vi "Open.vi"(8 "error in (no error)":errorcluster, 11 "UDP in":refnum<class "UDP.lvclass">) -> (0 "error out":errorcluster, 3 "UDP out":refnum<class "UDP.lvclass">)   [LabVIEW 2018, in "UDP.lvclass"]
doc: "Bus.lvclass:Open.vi\n\nThis is the template for the Open VI for the Bus class.\n\nInstrument Communication Module Version 1.0\nJuly, 2017 Original Code Consulting David Thomson\n www.originalcode.com"
uses:
  UDP.lvclass
  UDP.lvclass/UDP.ctl
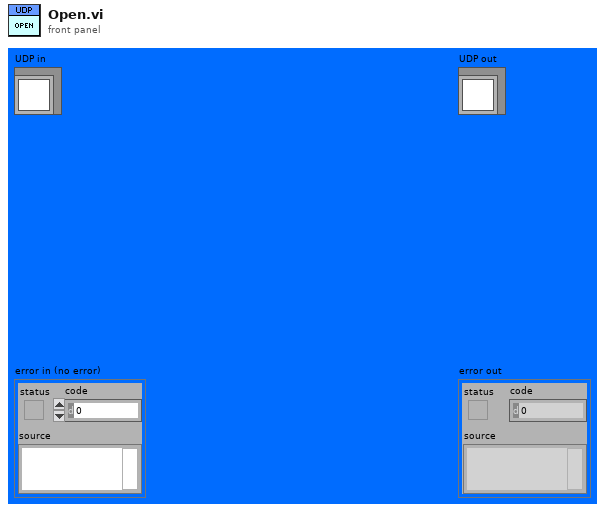
[diagram p1: front panel]
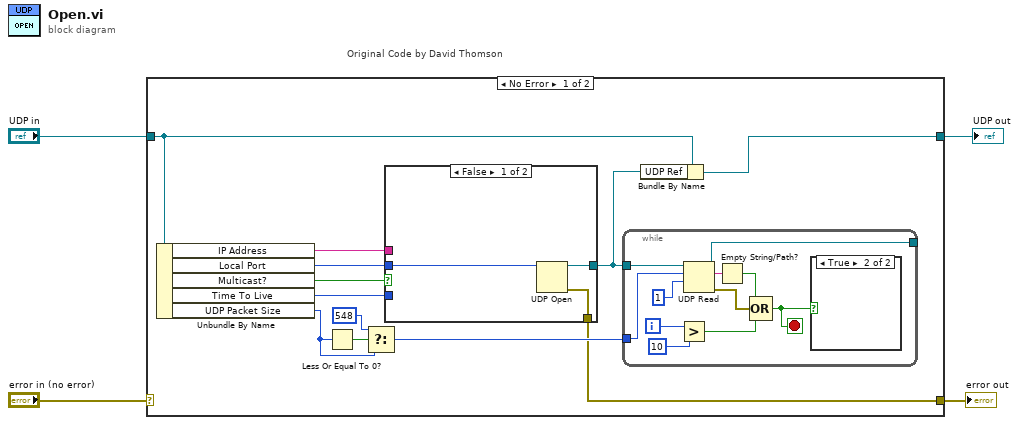
[diagram p0: block diagram]
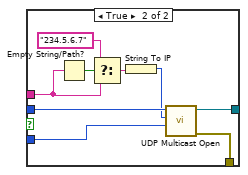
[diagram p2: hidden frame]
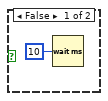
[diagram p3: hidden frame]
diagram:
  n1 = case "Original Code by David Thomson" shown="No Error" "error in (no error)" {
    selector: "error in (no error)" -> [_ w42]
    tunnel: [w11 w42] -> w1
    tunnel: [w6 w41] -> w2
    tunnel: "UDP in" -> [w7 w41]
    frame No Error {
      n2 = Unbundle By Name(w7) -> ("IP Address"=w9:string, "Local Port"=w16:u16, "Multicast?"=w10:bool, "Time To Live"=w8:u16, "UDP Packet Size"=w13:i32)
      n3 = Less Or Equal To 0?(x=w13) -> (x <= 0?=w15:bool)
      n4 = Select(t=548 ("max size (548)"), s=w15, f=w13) -> (s? t:f=w12:i32)
      n5 = case shown="False" w10 {
        tunnel: w16 -> [w19 w26]
        tunnel: [w18 w28] -> w5
        tunnel: [w17 w27] -> w11
        tunnel: w9 -> [_ w22]
        tunnel: w8 -> [_ w20]
        frame False {
          n6 = UDP Open(11:w19) -> (port=w18:refnum<k16>, 0:w17:errorcluster)  [unwired: 1 in, 4 out]
        }
        frame True {
          n7 = Empty String/Path?(string/path=w22) -> (empty?=w25:bool)
          n8 = Select(t="234.5.6.7", s=w25, f=w22) -> (s? t:f=w24:string)
          n9 = String To IP(1:w24) -> (0:w21:u32)
          n10 = call-poly "UDP Multicast Open.vi"("time-to-live (1)"=w20, "multicast addr"=w21, "port"=w26) -> ("error out"=w27:errorcluster, "connection ID"=w28:refnum<k16>)  [unwired: 6 in, 1 out]
        }
      }
      n11 = while {
        tunnel: w5 -> [w39]
        tunnel: [w36] -> _
        tunnel: w12 -> [w35]
        i -> [w32]
        stop <- w30 stop-if-true
        n12 = Greater?(x=w32, y=10) -> (0:w29:bool)
        n13 = UDP Read(connection ID=w39, max size (548)=w35, timeout ms (25000)=1) -> (data out=w37:string, error out=w33:errorcluster, 3:w36:refnum<k16>)  [unwired: 1 in, 2 out]
        n14 = Empty String/Path?(string/path=w37) -> (empty?=w34:bool)
        n15 = Compound Arithmetic op=OR(w34, w33, w29) -> (w30:bool)
        n16 = case shown="True" w30 {
          frame False {
            n17 = Wait (ms)(milliseconds to wait=u32 10) -> ()  [unwired: 1 out]
          }
          frame True {
          }
        }
      }
      n18 = Bundle By Name(cluster=w7, "UDP Ref"=w5) -> (w6:refnum<class "UDP.lvclass">)
    }
    frame Error {
    }
  }
  "error out" <- w1
  "UDP out" <- w2
